vi "Publish Alarm Screen.vi"(7 "LabVIEW Web Service Request":refnum<class "Web Request.lvclass">) -> ()   [LabVIEW 2018]
uses:
  <vilib>/wsapi/Web Request.lvclass
panel:
  # "Use the Web Service Request input terminal to call the VIs on the Web Services palette. Do not remove it from the connector pane unless you don't need access to the palette."
  # "Each additional control wired to the connector pane will be available as an input in the URL. To include an indicator in terminal-mode output (the default setting), it must also be wired to the connector pane."
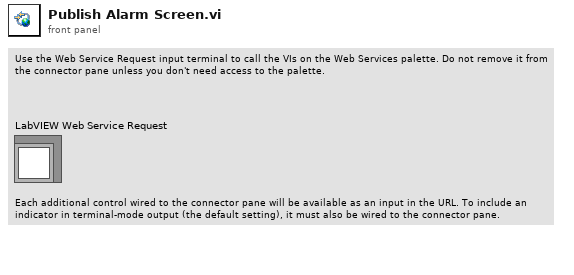
[diagram p1: front panel]
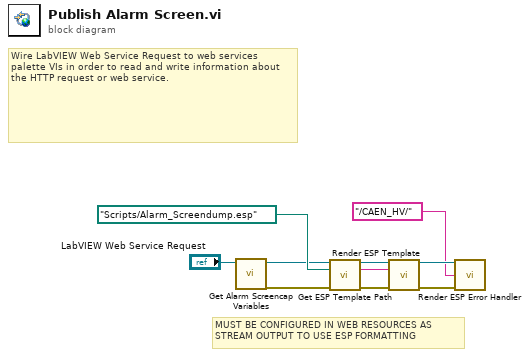
[diagram p0: block diagram]
diagram:
  # "MUST BE CONFIGURED IN WEB RESOURCES AS\nSTREAM OUTPUT TO USE ESP FORMATTING"
  # "Wire LabVIEW Web Service Request to web services palette VIs in order to read and write information about the HTTP request or web service."
  n1 = call "Get Alarm Screencap Variables.vi"("LabVIEW Web Service Request"="LabVIEW Web Service Request") -> ("error out"=w2:errorcluster, "LabVIEW Web Service Request out"=w3:refnum<class "Web Request.lvclass">)  [unwired: 9 in]
  n2 = call "Get ESP Template Path.vi"("LabVIEW Web Service Request"=w3, "Relative Template Path"=path "Scripts/Alarm_Screendump.esp", "error in (no error)"=w2) -> ("LabVIEW Web Service Request out"=w4:refnum<class "Web Request.lvclass">, "Template Name"=w6:string, "error out"=w7:errorcluster)  [unwired: 10 in]
  n3 = call <vilib>:"Render ESP Template.vi"("LabVIEW Web Service Request"=w4, "espName"=w6, "error in (no error)"=w7) -> ("LabVIEW Web Service Request out"=w9:refnum<class "Web Request.lvclass">, "error out"=w10:errorcluster)  [unwired: 11 in]
  n4 = call "Render ESP Error Handler.vi"("LabVIEW Web Service Request"=w9, "Link"="/CAEN_HV/", "error in (no error)"=w10) -> ()  [unwired: 11 in, 2 out]
